vi "Init_UI_Buttons.vi"(0 "VISAResourceName in":refnum<vi>, 2 "Bool Refnum 2":refnum<vi>, 3 "Bool Refnum":refnum<vi>, 5 "Str Refnum":refnum<vi>, 7 "DigNum Refnum":refnum<vi>, 9 "DigNum Refnum 2":refnum<vi>, 11 "error in (no error)":errorcluster, 12 "DigNum Refnum 3":refnum<vi>, 13 "Ring Refnum":refnum<vi>) -> (15 "error out":errorcluster)   [LabVIEW 2023, in "Arduino_TranslationStage_UI.lvlib" / "Arduino_Stepper.lvclass"]
uses:
  Arduino_Stepper.lvclass
  Arduino_Stepper.lvclass/Arduino_Stepper.ctl
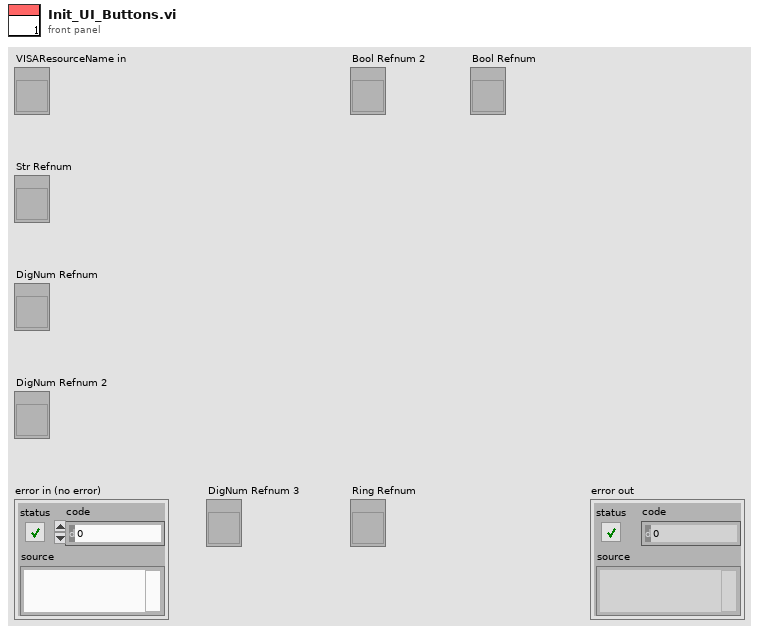
[diagram p1: front panel]
types:
  T1 = enum8{"Enabled", "Disabled", "Disabled and Grayed Out"}
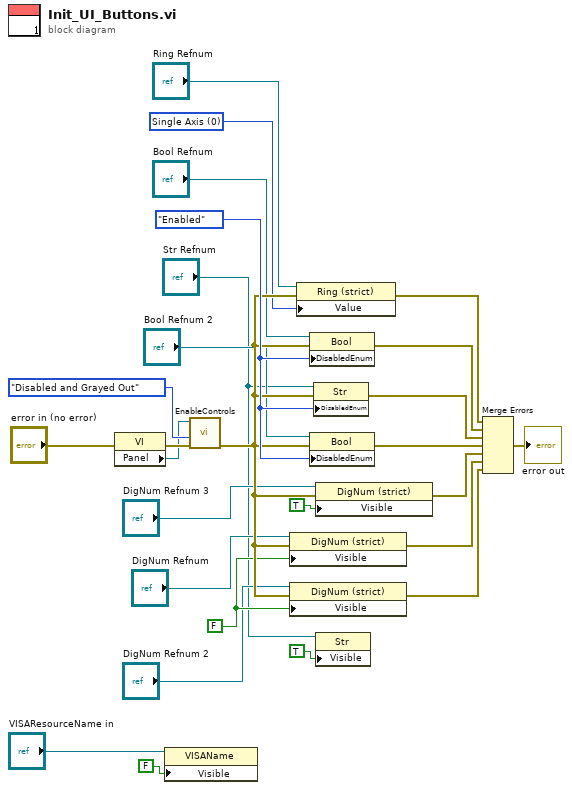
[diagram p0: block diagram]
diagram:
  w15 = 0 items=["Single Axis", "Raster"] ("Scan Mode")
  w14 = FALSE ("Visible")
  w25 = T1."Enabled" ("Disabled")
  n1 = property class="VI"(error in="error in (no error)") -> (error out=w12:errorcluster, "Panel"=w9:refnum<vi>)  [unwired: 1 in, 1 out]
  n2 = property on="Property Node" class="VISAName"(reference="VISAResourceName in", "Visible"=FALSE) -> ()  [unwired: 1 in, 2 out]
  n3 = call "EnableControls.vi"("error in (no error)"=w12, "Disabled"=T1."Disabled and Grayed Out", "Panel in"=w9) -> ("error out"=w24:errorcluster)  [unwired: 8 in]
  n4 = property on="Property Node" class="DigNum (strict)"(reference="DigNum Refnum", error in=w24, "Visible"=w14) -> (error out=w21:errorcluster)  [unwired: 1 out]
  n5 = property on="Property Node" class="DigNum (strict)"(reference="DigNum Refnum 2", error in=w24, "Visible"=w14) -> (error out=w22:errorcluster)  [unwired: 1 out]
  n6 = property on="Property Node" class="Ring (strict)"(reference="Ring Refnum", error in=w24, "Value"=w15) -> (error out=w16:errorcluster)  [unwired: 1 out]
  n7 = property on="Property Node" class="Bool"(reference="Bool Refnum", error in=w24, "DisabledEnum"=w25) -> (error out=w17:errorcluster)  [unwired: 1 out]
  n8 = property on="Property Node" class="Bool"(reference="Bool Refnum 2", error in=w24, "DisabledEnum"=w25) -> (error out=w19:errorcluster)  [unwired: 1 out]
  n9 = property on="Property Node" class="Str"(reference="Str Refnum", error in=w24, "DisabledEnum"=w25) -> (error out=w18:errorcluster)  [unwired: 1 out]
  n10 = property on="Property Node" class="DigNum (strict)"(reference="DigNum Refnum 3", error in=w24, "Visible"=TRUE) -> (error out=w20:errorcluster)  [unwired: 1 out]
  n11 = property on="Property Node" class="Str"(reference="Str Refnum", "Visible"=TRUE) -> ()  [unwired: 1 in, 2 out]
  n12 = Merge Errors(w16, w17, w18, w19, w20, w21, w22) -> (→"error out":errorcluster)
